vi "DifferentialStrictFollower Setter.vi"(0 "DeviceReference":T1, 3 "Update Frequency (Hz)":dbl=100.0, 5 "StopSendingOtherRequests":bool=TRUE, 7 "MasterID":i32) -> (4 "DeviceReference Out":T1)   [LabVIEW 2023]
doc: "Follow the differential motor output of another Talon while ignoring the master's invert setting.\nIf Talon is in torque control, the torque is copied - which will increase the total torque applied. If Talon is in percent supply output control, the duty cycle is matched. Motor direction is strictly determined by the configured invert and not the master. If you want motor direction to match or oppose the master, use FollowerRequest instead."
uses:
  Users/Cory/Documents/PhoenixPro-LabVIEW-Generation/controls/DeviceReference.ctl
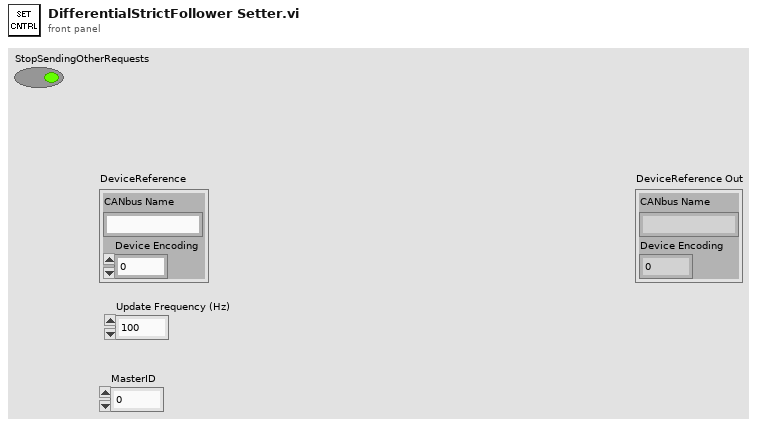
[diagram p1: front panel]
types:
  T1 = typedef "DeviceReference.ctl" = cluster{"CANbus Name":string, "Device Encoding":u32}
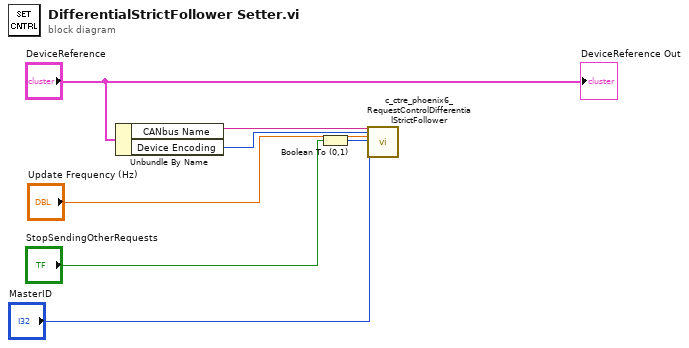
[diagram p0: block diagram]
diagram:
  n1 = Unbundle By Name("DeviceReference") -> ("CANbus Name"=w6:string, "Device Encoding"=w5:u32)
  n2 = Boolean To (0,1)(Boolean="StopSendingOtherRequests") -> (0, 1=w2:i16)
  n3 = call <vilib>:"c_ctre_phoenix6_RequestControlDifferentialStrictFollower.vi"("String 2"=w6, "Numeric 2"=w5, "Numeric 3"="Update Frequency (Hz)", "Numeric 4"=w2, "Numeric 5"="MasterID") -> ()  [unwired: 21 in, 2 out]
  "DeviceReference Out" <- "DeviceReference"
